vi "Singleton Core.vi"(7 "Action":enum16{"Init", "Write Object", "Read Object"}(ring), 8 "error in (no error)":errorcluster, 10 "Class in":refnum<class>) -> (0 "error out":errorcluster, 2 "Class out":refnum<class>)   [LabVIEW 2020, in "Singleton.lvlib"]
uses:
  Singleton.lvlib
  Singleton.lvclass
  Singleton.lvclass/Singleton.ctl
  <vilib>/ErrorRing/Error Ring.xnode
  <vilib>/Utility/error.llb/Error Cluster From Error Code.vi
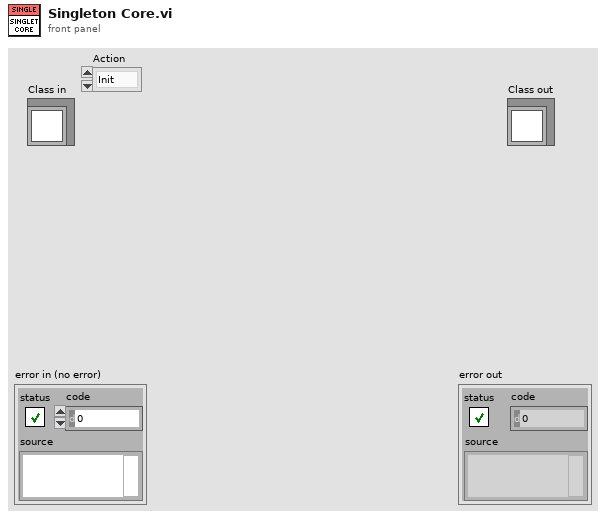
[diagram p1: front panel]
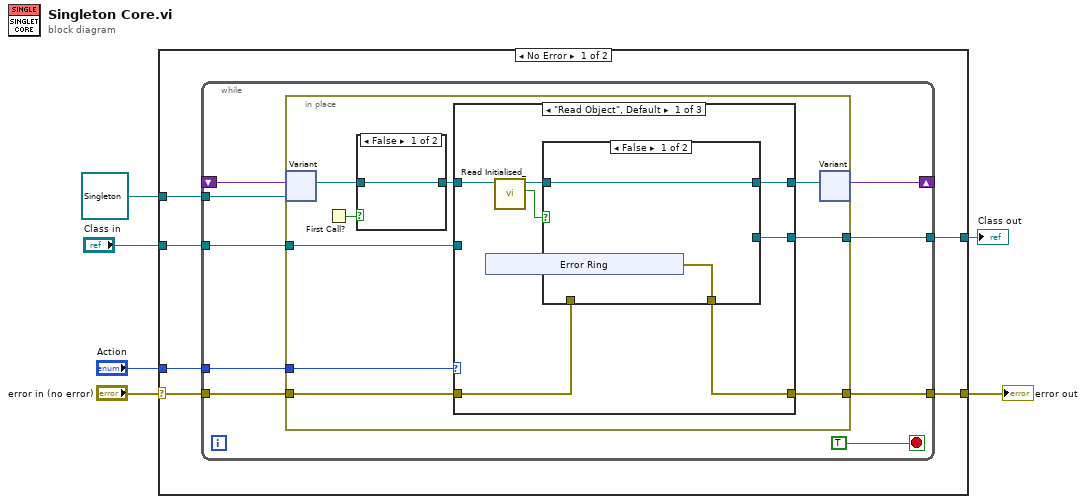
[diagram p0: block diagram]
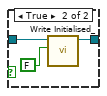
[diagram p2: hidden frame]
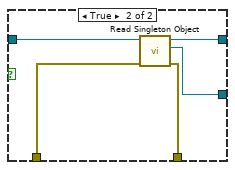
[diagram p3: hidden frame]
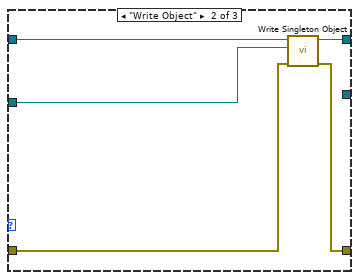
[diagram p4: hidden frame]
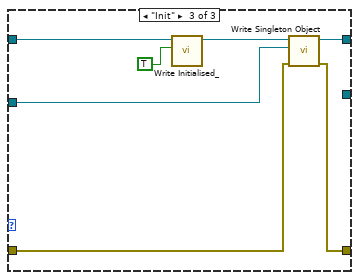
[diagram p5: hidden frame]
diagram:
  n1 = case shown="No Error" "error in (no error)" {
    selector: "error in (no error)" -> [w11 w66]
    tunnel: [w10 w66] -> w5
    tunnel: refnum<class "Singleton.lvclass"> refnum ("Singleton in") -> [w12 _]
    tunnel: "Class in" -> [w8 _]
    tunnel: "Action" -> [w9 _]
    tunnel: [w7 _] -> w1
    frame No Error {
      n2 = while {
        tunnel: w12 -> [w14]
        tunnel: w11 -> [w19]
        tunnel: [w18] -> w10
        shift-right: [w16] -> _
        shift-left: _ -> [w17]
        tunnel: w9 -> [w20]
        tunnel: w8 -> [w15]
        tunnel: [w13] -> w7
        stop <- TRUE stop-if-true
        n3 = in-place {
          in-place-border: w20 -> [w30]
          in-place-border: w19 -> [w29]
          in-place-border: w15 -> [w28]
          in-place-border: [w27] -> w18
          in-place-border: [w25] -> w13
          n4 = in-place-variant #1(w17, w14) -> (w24:refnum<class "Singleton.lvclass">)  [unwired: 1 out]
          n5 = First Call?() -> (First Call?: T/F=w22:bool)
          n6 = case shown="False" w22 {
            tunnel: w24 -> [w31 w34]
            tunnel: [w31 w33] -> w23
            frame False {
            }
            frame True {
              n7 = call "Write Initialised_.vi"("Initialised?"=FALSE, "Singleton in"=w34) -> ("Singleton out"=w33:refnum<class "Singleton.lvclass">)  [unwired: 8 in, 1 out]
            }
          }
          n8 = case shown="\"Read Object\", Default" w30 {
            tunnel: w23 -> [w37 w58 w60]
            tunnel: w29 -> [w39 w56 w63]
            tunnel: [w38 w55 w62] -> w27
            tunnel: w28 -> [_ w57 w64]
            tunnel: [w41 w54 w65] -> w26
            tunnel: [w40 _ _] -> w25
            frame "Read Object", Default {
              n9 = call "Read Initialised_.vi"("Singleton in"=w37) -> ("Initialised?"=w35:bool, "Singleton out"=w36:refnum<class "Singleton.lvclass">)  [unwired: 8 in, 1 out]
              n10 = case shown="False" w35 {
                tunnel: [w43 w53] -> w41
                tunnel: [_ w52] -> w40
                tunnel: w39 -> [_ w51]
                tunnel: [w42 w50] -> w38
                tunnel: w36 -> [w43 w49]
                frame False {
                  n11 = xnode "Error Ring"() -> ("error out"=w42:errorcluster)
                }
                frame True {
                  n12 = call "Read Singleton Object.vi"("error in (no error)"=w51, "Singleton in"=w49) -> ("error out"=w50:errorcluster, "Singleton Object"=w52:refnum<class>, "Singleton out"=w53:refnum<class "Singleton.lvclass">)  [unwired: 7 in]
                }
              }
            }
            frame "Write Object" {
              n13 = call "Write Singleton Object.vi"("error in (no error)"=w56, "Singleton Object"=w57, "Singleton in"=w58) -> ("error out"=w55:errorcluster, "Singleton out"=w54:refnum<class "Singleton.lvclass">)  [unwired: 7 in]
            }
            frame "Init" {
              n14 = call "Write Initialised_.vi"("Initialised?"=TRUE, "Singleton in"=w60) -> ("Singleton out"=w61:refnum<class "Singleton.lvclass">)  [unwired: 8 in, 1 out]
              n15 = call "Write Singleton Object.vi"("error in (no error)"=w63, "Singleton Object"=w64, "Singleton in"=w61) -> ("error out"=w62:errorcluster, "Singleton out"=w65:refnum<class "Singleton.lvclass">)  [unwired: 7 in]
            }
          }
          n16 = in-place-variant #1(w26) -> (w16:variant)  [unwired: 1 out]
        }
      }
    }
    frame Error {
    }
  }
  "error out" <- w5
  "Class out" <- w1
